vi "FindColumnName V2_0.vi"(0 "Columns":string[](array[string]), 5 "start cell in":cluster{"row":i32, "column":i32}, 9 "Column Name":string, 11 "error in (no error)":errorcluster) -> (6 "start cell out":cluster{"row":i32, "column":i32}, 15 "error out":errorcluster)   [LabVIEW 2015]
doc: "This vi will search the array of column headers to find the index of the disired column\nit will then put that number in the start cell out cluster"
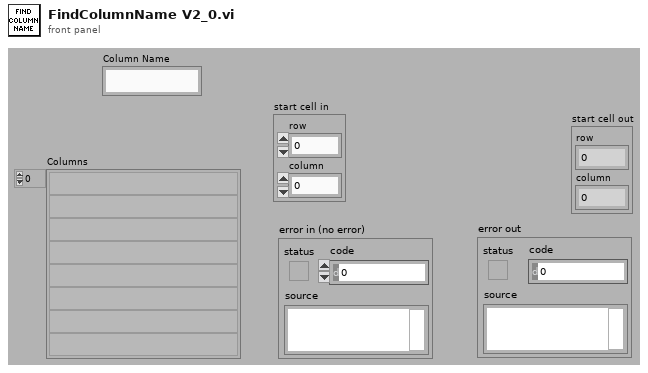
[diagram p1: front panel]
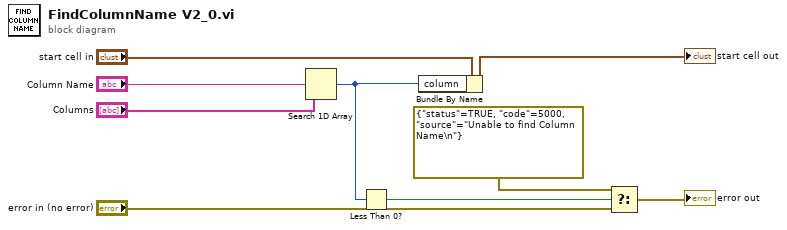
[diagram p0: block diagram]
diagram:
  n1 = Search 1D Array(1D array="Columns", element="Column Name") -> (index of element=w6:i32)  [unwired: 1 in]
  n2 = Less Than 0?(x=w6) -> (x < 0?=w3:bool)
  n3 = Bundle By Name(cluster="start cell in", "column"=w6) -> (→"start cell out":cluster{"row":i32, "column":i32})
  n4 = Select(t=errorcluster {"status"=TRUE, "code"=5000, "source"="Unable to find Column Name\n"}, s=w3, f="error in (no error)") -> (s? t:f=→"error out":errorcluster)
